vi "Diagnostic Measurement.vi"(8 "error in (no error)":errorcluster, 11 "MSX-E3701 in":refnum<class "MSX-E3701.lvclass">) -> (0 "error out":errorcluster, 3 "MSX-E3701 out":refnum<class "MSX-E3701.lvclass">)   [LabVIEW 2014, in "MSX-E3701.lvlib" / "MSX-E3701.lvclass"]
doc: "En base a los datos de promedio de los transductores el código analiza si el transductor está cortado o sin conectar."
uses:
  MSX-E3701.lvclass
  MSX-E3701.lvclass/MSX-E3701.ctl
  DriverMasterSync/build/DriverMasterSync.lvlibp/Modules/HAL/DriverMasterSync/DriverMasterSyncClass/DriverMasterSync.lvclass
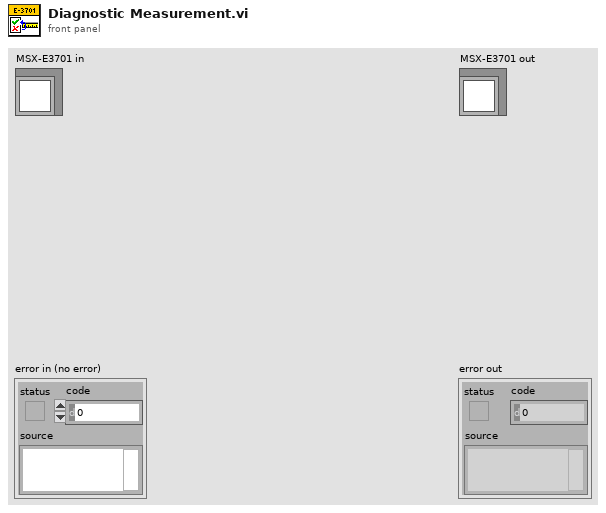
[diagram p1: front panel]
types:
  T1 = typedef "DriverMasterSync.lvlibp/HAL Config Data.ctl" = cluster{"HWSync Index":u32, "Driver Name":string, "Channel Mask":u64}
  T2 = typedef "DriverMasterSync.lvlibp/WINFAS 2 Data Queue.lvlib/Acquisition Data Cluster.ctl" = T3[]
  T3 = typedef "DriverMasterSync.lvlibp/WINFAS 2 Data Queue.lvlib/Acquisition Data 1 Sample Cluster.ctl" = cluster{"TDX":sgl[], "Encoder":sgl}
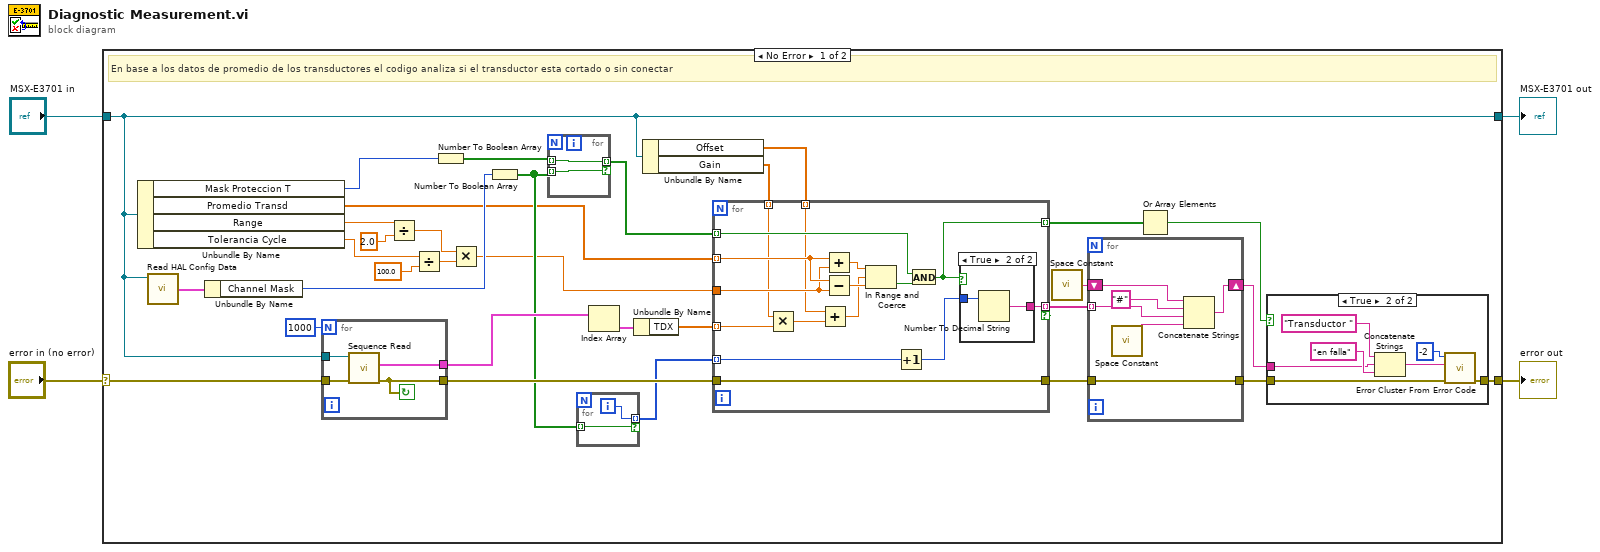
[diagram p0: block diagram]
diagram:
  n1 = case shown="No Error" "error in (no error)" {
    selector: "error in (no error)" -> [w35 w78]
    tunnel: [w32 w78] -> w4
    tunnel: [w7 w77] -> w3
    tunnel: "MSX-E3701 in" -> [w7 w77]
    frame No Error {
      # "En base a los datos de promedio de los transductores el codigo analiza si el transductor esta cortado o sin conectar"
      n2 = Unbundle By Name(w7) -> ("Mask Proteccion T"=w33:u64, "Promedio Transd"=w15:sgl[], "Range"=w9:sgl, "Tolerancia Cycle"=w8:sgl)
      n3 = call "Read HAL Config Data.vi"("DriverMasterSync in"=w7) -> ("HAL Config Data"=w23:T1)  [unwired: 8 in, 2 out]
      n4 = Unbundle By Name(w23) -> ("Channel Mask"=w22:u64)
      n5 = for {
        N: 1000 -> [_]
        tunnel: [w42] -> w21
        tunnel: w35 -> [w41]
        tunnel: [w40] -> w34
        tunnel: w7 -> [w39]
        stop <- w40 continue-if-true
        n6 = call-dynamic "Sequence Read.vi"("error in (no error)"=w41, "MSX-E3701 in"=w39) -> ("error out"=w40:errorcluster, "Acquisition Data"=w42:T2)  [unwired: 6 in, 2 out]
      }
      n7 = Divide(x=w9, y=sgl 2.0) -> (x/y=w11:sgl)
      n8 = Divide(x=w8, y=sgl 100.0) -> (x/y=w36:sgl)
      n9 = Number To Boolean Array(number=w33) -> (Boolean array=w18:bool[])
      n10 = Multiply(x=w11, y=w36) -> (x*y=w14:sgl)
      n11 = Number To Boolean Array(number=w22) -> (Boolean array=w17:bool[])
      n12 = for {
        tunnel: w18 -> [w44] mode=indexing
        tunnel: [w44] -> w24 mode=indexing if=w43
        tunnel: w17 -> [w43] mode=indexing
      }
      n13 = for {
        tunnel: w17 -> [w37] mode=indexing
        tunnel: [w38] -> w16 mode=indexing if=w37
        i -> [w38]
      }
      n14 = Index Array(array=w21) -> (element=w20:T3)  [unwired: 1 in]
      n15 = Unbundle By Name(w20) -> ("TDX"=w19:sgl[])
      n16 = Unbundle By Name(w7) -> ("Offset"=w5:sgl[], "Gain"=w6:sgl[])
      n17 = for {
        tunnel: w34 -> [w74]
        tunnel: w24 -> [w71] mode=indexing
        tunnel: [w74] -> w28
        tunnel: [w70] -> w31 mode=indexing
        tunnel: [w72] -> w26 mode=indexing if=w70
        tunnel: w19 -> [w61] mode=indexing
        tunnel: w16 -> [w68] mode=indexing
        tunnel: w15 -> [w67] mode=indexing
        tunnel: w14 -> [w66]
        tunnel: w6 -> [w60] mode=indexing
        tunnel: w5 -> [w59] mode=indexing
        n18 = Multiply(x=w60, y=w61) -> (x*y=w63:sgl)
        n19 = Add(x=w59, y=w63) -> (x+y=w62:sgl)
        n20 = Add(x=w67, y=w66) -> (x+y=w65:sgl)
        n21 = Subtract(x=w67, y=w66) -> (x-y=w64:sgl)
        n22 = In Range and Coerce(upper limit=w65, x=w62, lower limit=w64) -> (In Range?=w73:bool)  [unwired: 1 out]
        n23 = Increment(x=w68) -> (x+1=w69:i32)
        n24 = And(x=w71, y=w73) -> (x .and. y?=w70:bool)
        n25 = case shown="True" w70 {
          tunnel: w69 -> [_ w76]
          tunnel: [_ w75] -> w72
          frame False {
          }
          frame True {
            n26 = Number To Decimal String(number=w76) -> (decimal integer string=w75:string)  [unwired: 1 in]
          }
        }
      }
      n27 = call <vilib>:"Space Constant.vi"() -> ("String"=w27:string)
      n28 = for {
        tunnel: [w50] -> w29
        tunnel: w28 -> [w50]
        shift-right: [w49] -> w25
        shift-left: w27 -> [w48]
        tunnel: w26 -> [w46] mode=indexing
        n29 = call <vilib>:"Space Constant.vi"() -> ("String"=w45:string)
        n30 = Concatenate Strings(w48, "#" ("string"), w46, w45) -> (w49:string)
      }
      n31 = Or Array Elements(Boolean array=w31) -> (logical OR=w30:bool)
      n32 = case shown="True" w30 {
        tunnel: w29 -> [w51 w54]
        tunnel: [w51 w53] -> w32
        tunnel: w25 -> [_ w52]
        frame False {
        }
        frame True {
          n33 = Concatenate Strings("Transductor ", w52, "en falla" ("string")) -> (w55:string)
          n34 = call <vilib>:"Error Cluster From Error Code.vi"("error in (no error)"=w54, "error message (\"\")"=w55, "error code (0)"=-2) -> ("error out"=w53:errorcluster)  [unwired: 6 in]
        }
      }
    }
    frame Error {
    }
  }
  "error out" <- w4
  "MSX-E3701 out" <- w3
